vi "extract_fft_components.vi"(6 "Freq resolution":dbl, 7 "High cutoff":sgl=inf, 9 "Cycles in block":i32, 10 "Components":T1, 11 "FFT {X} in":cdb[](array[numeric])) -> (3 "FFT {X} out":cdb[](array[numeric]))   [LabVIEW 2012]
panel:
  # "Process an FFT spectrum to extract FFT and harmonics with respect to a particular coherently sampled signal.  What this means in practice is zeroing out selected bins that don't contain the desired signal.  This operates on the full FFT result block, preserving the redundant conjugate structure of the two halves, which is useful if we are going to do an inverse FFT. \n\n\"High cutoff\" is optional, and \"Freq resolution\" is only needed when it is specified."
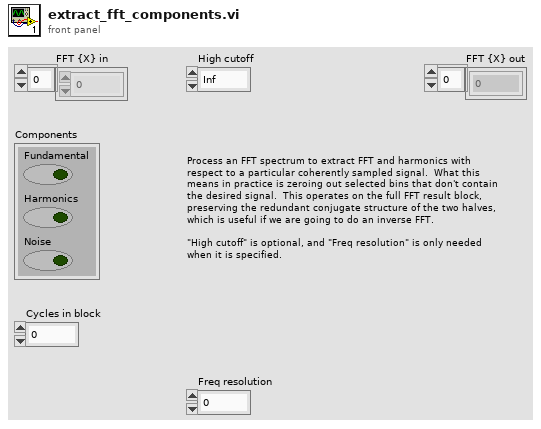
[diagram p1: front panel]
types:
  T1 = cluster{"Fundamental":bool, "Harmonics":bool, "Noise":bool}
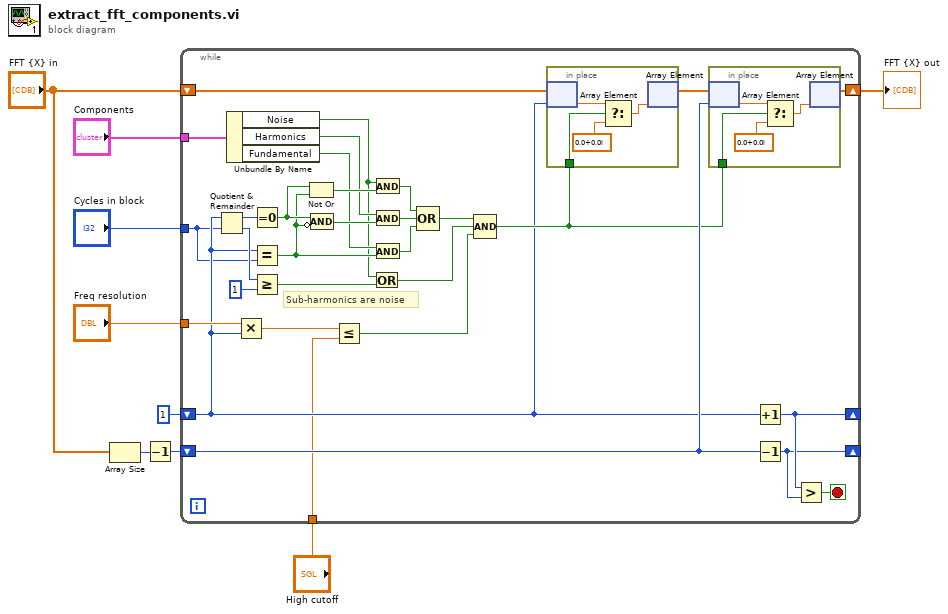
[diagram p0: block diagram]
diagram:
  n1 = Array Size(array="FFT {X} in") -> (size(s)=w2:i32)
  n2 = Decrement(x=w2) -> (x-1=w1:i32)
  n3 = while {
    shift-right: [w39] -> _
    shift-left: 1 -> [w12]
    shift-right: [w38] -> _
    shift-left: w1 -> [w32]
    tunnel: "Cycles in block" -> [w11]
    tunnel: "Components" -> [w35]
    shift-right: [w23] -> w7
    shift-left: "FFT {X} in" -> [w34]
    tunnel: "Freq resolution" -> [w15]
    tunnel: "High cutoff" -> [w10]
    stop <- w40 stop-if-true
    # "Sub-harmonics are noise"
    n4 = Quotient & Remainder(x=w12, y=w11) -> (x-y*floor(x/y)=w37:i32, floor(x/y)=w21:i32)
    n5 = Unbundle By Name(w35) -> ("Noise"=w22:bool, "Harmonics"=w30:bool, "Fundamental"=w28:bool)
    n6 = Multiply(x=w15, y=w12) -> (x*y=w14:dbl)
    n7 = Equal To 0?(x=w37) -> (x = 0?=w36:bool)
    n8 = Equal?(x=w12, y=w11) -> (x = y?=w27:bool)
    n9 = Greater Or Equal?(x=w21, y=1) -> (x >= y?=w19:bool)
    n10 = Not Or(1:w27, 2:w36) -> (0:w31:bool)
    n11 = Compound Arithmetic op=AND(w36, invert w27) -> (w29:bool)
    n12 = Less Or Equal?(x=w14, y=w10) -> (x <= y?=w13:bool)
    n13 = Or(x=w22, y=w19) -> (x .or. y?=w18:bool)
    n14 = And(x=w22, y=w31) -> (x .and. y?=w26:bool)
    n15 = And(x=w30, y=w29) -> (x .and. y?=w25:bool)
    n16 = And(x=w28, y=w27) -> (x .and. y?=w24:bool)
    n17 = Compound Arithmetic op=OR(w26, w25, w24) -> (w17:bool)
    n18 = Compound Arithmetic op=AND(w17, w18, w13) -> (w16:bool)
    n19 = in-place {
      in-place-border: w16 -> [w45]
      n20 = in-place-array #1(w34, w12) -> (w48:cdb)
      n21 = Select(t=w48, s=w45, f=cdb 0.0+0.0i) -> (s? t:f=w47:cdb)
      n22 = in-place-array #1(w47) -> (w33:cdb[])  [unwired: 1 out]
    }
    n23 = in-place {
      in-place-border: w16 -> [w41]
      n24 = in-place-array #2(w33, w32) -> (w44:cdb)
      n25 = Select(t=w44, s=w41, f=cdb 0.0+0.0i) -> (s? t:f=w43:cdb)
      n26 = in-place-array #2(w43) -> (w23:cdb[])  [unwired: 1 out]
    }
    n27 = Increment(x=w12) -> (x+1=w39:i32)
    n28 = Decrement(x=w32) -> (x-1=w38:i32)
    n29 = Greater?(x=w39, y=w38) -> (0:w40:bool)
  }
  "FFT {X} out" <- w7
